vi "CLUSTER CONCEPT.vi"() -> ()   [LabVIEW 2018]
panel:
  out "output cluster":T1
  out "output cluster 2":cluster{"sl.no":dbl, "ATTENDANCE ":bool, string}
  in  "Cluster":T1
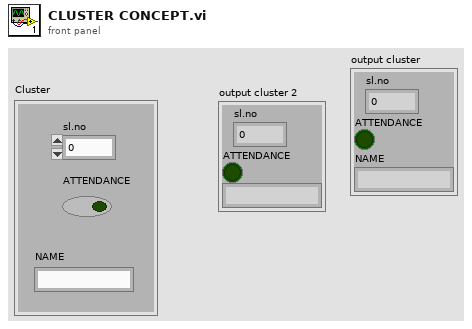
[diagram p1: front panel]
types:
  T1 = cluster{"sl.no":dbl, "ATTENDANCE ":bool, "NAME":string}
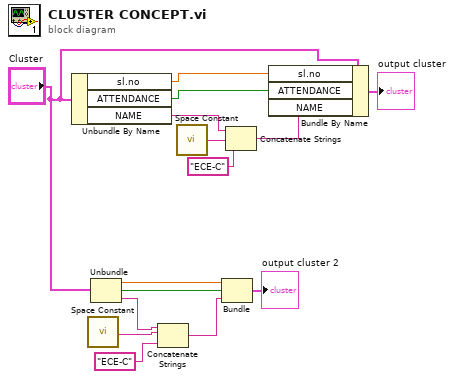
[diagram p0: block diagram]
diagram:
  n1 = Unbundle By Name("Cluster") -> ("sl.no"=w4:dbl, "ATTENDANCE"=w3:bool, "NAME"=w15:string)
  n2 = call <vilib>:"Space Constant.vi"() -> ("String"=w7:string)
  n3 = Unbundle("Cluster") -> ("sl.no"=w11:dbl, "ATTENDANCE"=w10:bool, "NAME"=w8:string)
  n4 = Concatenate Strings(w8, w7, "ECE-C") -> (w9:string)
  n5 = call <vilib>:"Space Constant.vi"() -> ("String"=w14:string)
  n6 = Bundle("sl.no"=w11, "ATTENDANCE"=w10, w9) -> (→"output cluster 2":cluster{"sl.no":dbl, "ATTENDANCE ":bool, string})  [unwired: 1 in]
  n7 = Concatenate Strings(w15, w14, "ECE-C") -> (w12:string)
  n8 = Bundle By Name(cluster="Cluster", "sl.no"=w4, "ATTENDANCE"=w3, "NAME"=w12) -> (→"output cluster":T1)
